vi "F.vi"() -> ()   [LabVIEW 2014]
panel:
  in  "F":dbl
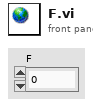
[diagram p1: front panel]
diagram:
